vi "SerialUntra.vi"(8 "Cluster":T1, 10 "cluster":T2) -> (1 "OUTPUT":T1)   [LabVIEW 2017, in "libVariable.lvlib" / "LibFunction.lvlib"]
uses:
  LibFunction.lvlib
  controls/QueueControl.ctl
  controls/CommandQueue.ctl
  <vilib>/Platform/TimedLoop/XDataNode/timing_clust.ctl
  <vilib>/Platform/TimedLoop/XDataNode/nitl_modes.ctl
  <vilib>/Platform/TimedLoop/XDataNode/wakeup.ctl
  mWorkToolkit/libSerial/STATEUART.ctl
  controls/state_board_control.ctl
  mWorkToolkit/libSerial/stateSerialUltra.ctl
  <vilib>/Instr/_visa.llb/VISA Flush IO Buffer Mask.ctl
  global/GLOBAL_STATE.vi
  <vilib>/Platform/TimedLoop/XDataNode/XDataNode.xnode
  <vilib>/Platform/TimedLoop/XDataNode/XDNodeRunTimeDep.lvlib
panel:
  out "Data Write":string
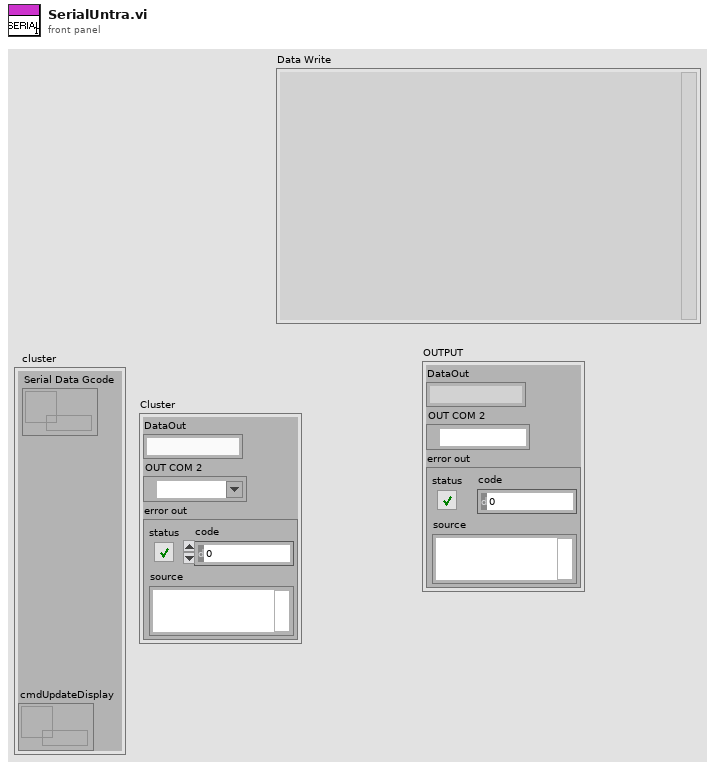
[diagram p1: front panel]
types:
  T1 = cluster{"DataOut":string, "OUT COM 2":refnum<visa-resource-name>, "error out":errorcluster}
  T2 = typedef "QueueControl.ctl" = cluster{"Serial Data Gcode":refnum<queue>, "cmdUpdateDisplay":refnum<queue>}
  T3 = typedef "STATEUART.ctl" = enum16{"INIT", "WRITE", "READ", "CHECKDATA", "IDLE", "STOP"}
  T4 = typedef "XDNodeRunTimeDep.lvlib/timing_clust.ctl" = cluster{"Expected End [f-1]":u64, "Actual End [f-1]":u64, "Finished Late? [f-1]":bool, "Expected End [i-1]":u64, "Actual End [i-1]":u64, "Finished Late? [i-1]":bool, "Expected Start [i]":u64, "Actual Start [i]":u64, "Expected Start [f]":u64, "Actual Start [f]":u64, "Source Name":string, "Structure Name":string, "Period":i64, "Deadline":i64, "Offset":i64, "Start":i64, "Priority":i32, "Timeout":i32, "Mode":T5, "Wakeup Reason":T6, "Error":errorcluster, "Source Type":string, "Secondary Source Type":string, "Global End Time":u64, "Global Start Time":u64, "Frame Duration":u64, "Iteration Duration":u64, "Assigned CPU":i32, "I/O Scan Engine Mode":u32}
  T5 = typedef "XDNodeRunTimeDep.lvlib/nitl_modes.ctl" = enum32{"No Change", "Process missed periods, maintain original phase", "Discard missed periods, maintain original phase", "Process missed periods, ignore original phase", "Discard missed periods, ignore original phase"}
  T6 = typedef "XDNodeRunTimeDep.lvlib/wakeup.ctl" = enum32{"Normal", "Aborted", "Asynchronous wakeup", "Timing source error", "Timed loop error", "Timeout"}
  T7 = typedef "state_board_control.ctl" = enum16{"Running", "Waiting", "Pos", "IDLE"}
  T8 = typedef "stateSerialUltra.ctl" = enum16{"findCOM", "Init", "CheckConnect", "Read", "Write", "exit"}
  T9 = cluster{"DataOut":string, "OUT COM 3":refnum<visa-resource-name>, "error out":errorcluster}
  T10 = cluster{string, "OUT COM 2":refnum<visa-resource-name>, "error IO":errorcluster}
  T11 = cluster{"DataOut":string, "OUT COM 2":refnum<visa-resource-name>, "error out\n":errorcluster}
  T12 = typedef "STATE_MK4DUERETURNSTATE.ctl" = enum16{"Pos", "Config", "Echo", "OK", "Step", "Error"}
  T13 = cluster{"OUTCONFIG":cluster{"StateMcodeConfig":enum16{"M203", "M201", "M92", "M3001"}, "X":dbl, "Y":dbl, "Z":dbl}, "outPOS":cluster{"StatePos":enum16{"Running", "Waiting", "Pos", "IDLE"}, "X":dbl, "Z":dbl, "Y":dbl, "A":dbl, "B":dbl}}
  T14 = cluster{"StateMcodeConfig":enum16{"M203", "M201", "M92", "M3001"}, "X":dbl, "Y":dbl, "Z":dbl}
  T15 = cluster{"StatePos":enum16{"Running", "Waiting", "Pos", "IDLE"}, "X":dbl, "Z":dbl, "Y":dbl, "A":dbl, "B":dbl}
  T16 = cluster{"StatePos":enum16{"Running", "Waiting", "Pos", "IDLE"}, "X":dbl, "Z":dbl, "Y":dbl}
  T17 = typedef "VISA Flush IO Buffer Mask.ctl" = u16
  T18 = cluster{"TIMEOUT_CONNECT":u32, "TIMEOUT_SENDCHECK":u32}
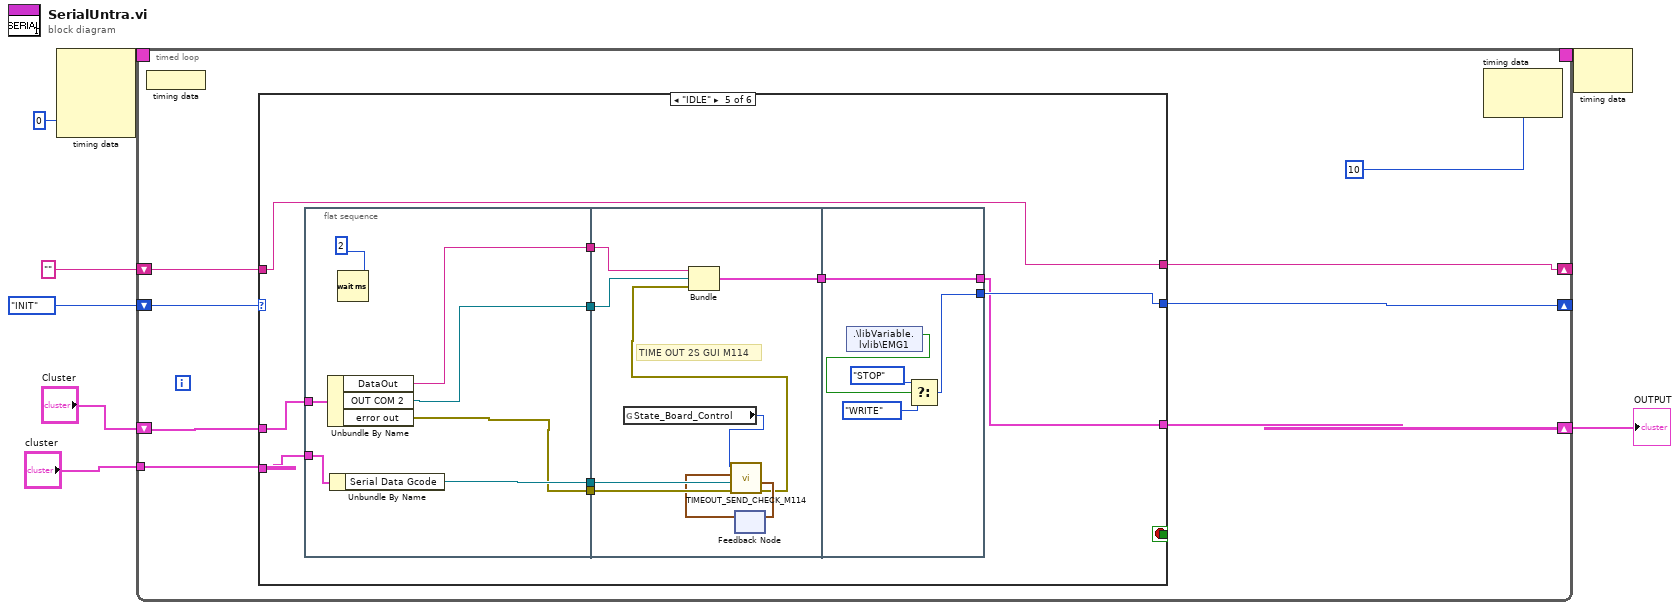
[diagram p0: block diagram]
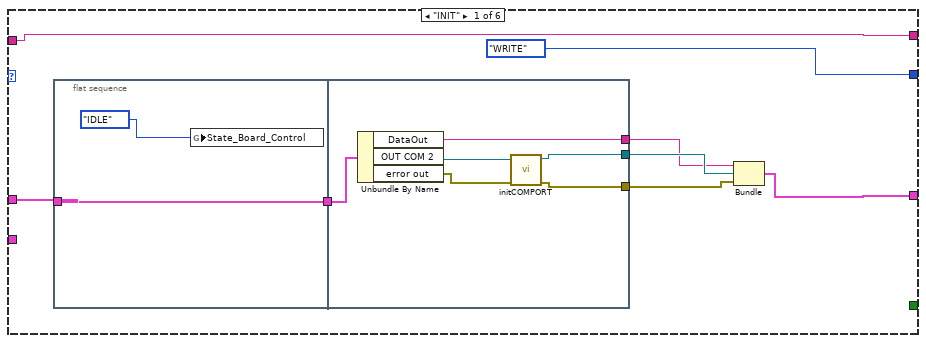
[diagram p2: hidden frame]
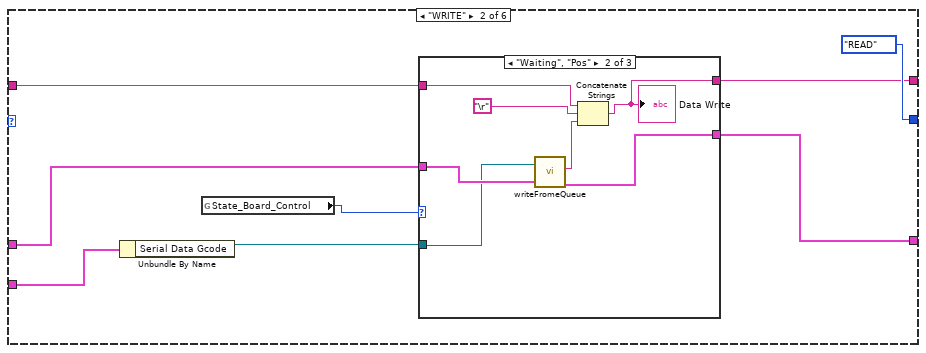
[diagram p3: hidden frame]
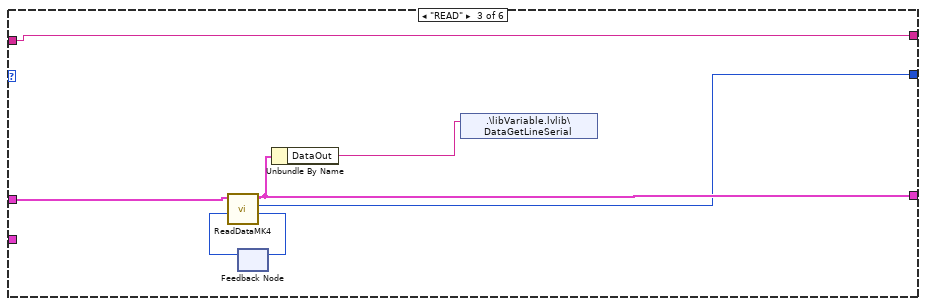
[diagram p6: hidden frame]
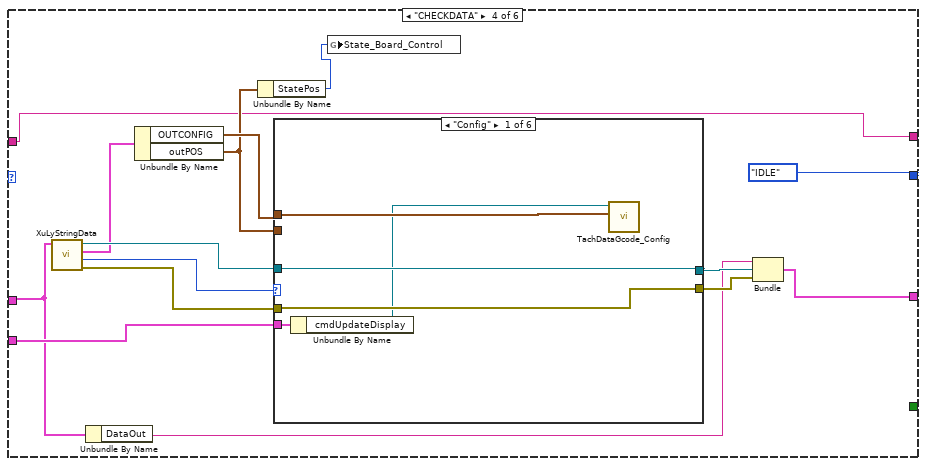
[diagram p7: hidden frame]
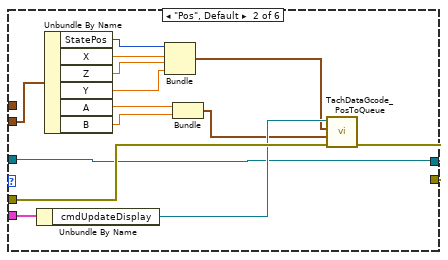
[diagram p8: hidden frame]
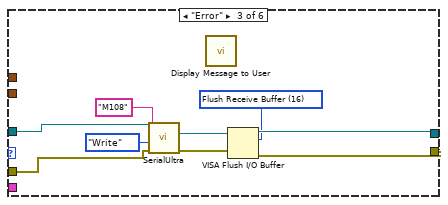
[diagram p9: hidden frame]
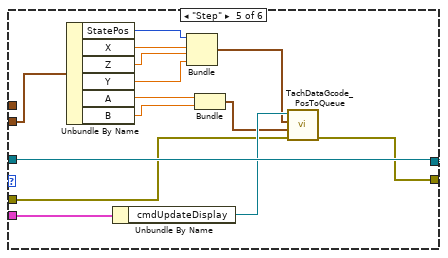
[diagram p11: hidden frame]
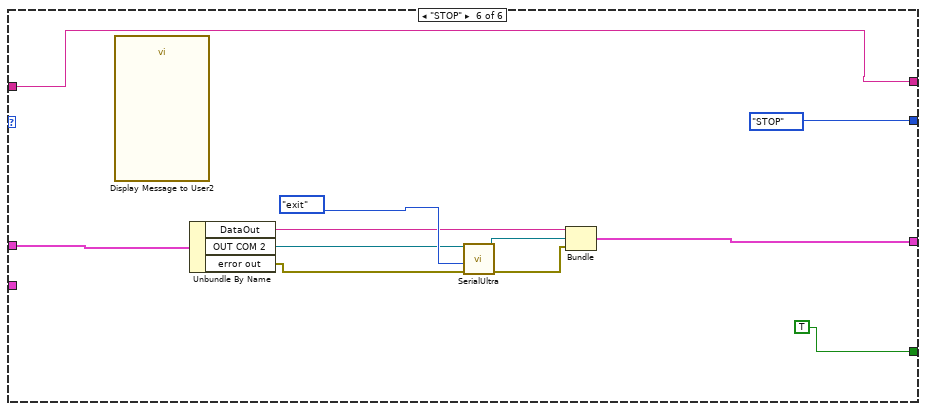
[diagram p13: hidden frame]
diagram:
  n1 = node-c288(0 ("Processor")) -> (w8:T4)  [unwired: 3 in]
  n2 = timed-loop {
    shift-right: [w14] -> _
    shift-left: STATEUART."INIT" -> [w17]
    shift-right: [w13] -> w2
    shift-left: "Cluster" -> [w15]
    timing: w8 -> [_]
    timing-out: [_] -> w7
    tunnel: "cluster" -> [w16]
    shift-right: [w9] -> _
    shift-left: "" -> [w10]
    stop <- w11 stop-if-true
    n3 = node-c288() -> ()  [unwired: 1 in]
    n4 = case shown="\"IDLE\"" w17 {
      tunnel: [STATEUART."WRITE" STATEUART."READ" w54 STATEUART."IDLE" w125 STATEUART."STOP"] -> w14
      tunnel: w15 -> [w22 w40 w59 w63 w130 w155]
      tunnel: [w20 w38 w56 w64 w123 w154] -> w13
      tunnel: w16 -> [_ w41 _ w68 w122 _]
      tunnel: [_ _ _ _ _ TRUE] -> w11
      tunnel: w10 -> [w18 w36 w53 w61 w121 w152]
      tunnel: [w18 w35 w53 w61 w121 w152] -> w9
      frame "INIT" {
        n5 = flat-sequence {
          tunnel: [w27] -> w25
          tunnel: w22 -> [w27]
          tunnel: w25 -> [w30]
          tunnel: [w31] -> w19
          tunnel: [w29] -> w23
          tunnel: [w28] -> w24
          frame #0 {
            n6 = global write "GLOBAL_STATE.vi" "State_Board_Control"(state_board_control."IDLE" ("state_board_STM1")) -> ()
          }
          frame #1 {
            n7 = Unbundle By Name(w30) -> ("DataOut"=w31:string, "OUT COM 2"=w33:refnum<visa-resource-name>, "error out"=w32:errorcluster)
            n8 = call "initCOMPORT.vi"("error IO"=w32, "OUT COM 2"=w33) -> ("error out"=w29:errorcluster, "OUT COM 3"=w28:refnum<visa-resource-name>)  [unwired: 8 in]
          }
        }
        n9 = Bundle("DataOut"=w19, "OUT COM 3"=w24, "error out"=w23) -> (w20:T9)  [unwired: 1 in]
      }
      frame "WRITE" {
        n10 = Unbundle By Name(w41) -> ("Serial Data Gcode"=w39:refnum<queue>)
        n11 = global read "GLOBAL_STATE.vi" "State_Board_Control"() -> (w34:T7)
        n12 = case shown="\"Waiting\", \"Pos\"" w34 {
          tunnel: w40 -> [w43 w50 w52]
          tunnel: w39 -> [_ w49 _]
          tunnel: [w43 w48 w52] -> w38
          tunnel: w36 -> [w42 w47 w51]
          tunnel: [w42 w46 w51] -> w35
          frame "Running", Default {
          }
          frame "Waiting", "Pos" {
            n13 = call "writeFromeQueue.vi"("queue"=w49, "Cluster"=w50) -> ("output cluster"=w48:T10, "Data Write"=w45:string)  [unwired: 7 in, 1 out]
            n14 = Concatenate Strings(w47, "\r", w45) -> (w46:string)
            "Data Write" <- w46
          }
          frame "IDLE" {
          }
        }
      }
      frame "READ" {
        n15 = feedback #1() -> (w57:u32)  [unwired: 1 in]
        n16 = call "ReadDataMK4.vi"("millisecondIN"=w57, "input cluster"=w59) -> ("millisecondOUT"=w58:u32, "STATEUART"=w54:T3, "Cluster"=w56:T11)  [unwired: 7 in]
        n17 = feedback-in #1(w58) -> ()
        n18 = Unbundle By Name(w56) -> ("DataOut"=w55:string)
        n19 = shared-variable ".\\libVariable.lvlib\\DataGetLineSerial"(w55) -> ()  [unwired: 1 in, 1 out]
      }
      frame "CHECKDATA" {
        n20 = call "XuLyStringData.vi"("input cluster"=w63) -> ("error out"=w69:errorcluster, "Return State"=w70:T12, "output cluster 2"=w65:T13, "OUT COM 2"=w71:refnum<visa-resource-name>)  [unwired: 3 in]
        n21 = Unbundle By Name(w63) -> ("DataOut"=w62:string)
        n22 = Unbundle By Name(w65) -> ("OUTCONFIG"=w67:T14, "outPOS"=w66:T15)
        n23 = Unbundle By Name(w66) -> ("StatePos"=w60:enum16{"Running", "Waiting", "Pos", "IDLE"})
        n24 = case shown="\"Config\"" w70 {
          tunnel: [w76 w91 w96 w103 w114 w119] -> w73
          tunnel: w69 -> [w76 w92 w94 w103 w115 w119]
          tunnel: w71 -> [w78 w89 w102 w104 w118 w120]
          tunnel: [w78 w89 w97 w104 w118 w120] -> w72
          tunnel: w68 -> [w77 w93 _ _ w117 _]
          tunnel: w67 -> [w79 _ _ _ _ _]
          tunnel: w66 -> [_ w88 _ _ w108 _]
          frame "Config" {
            n25 = Unbundle By Name(w77) -> ("cmdUpdateDisplay"=w75:refnum<queue>)
            n26 = call "TachDataGcode_Config.vi"("OUTCONFIG"=w79, "queue out"=w75) -> ()  [unwired: 10 in]
          }
          frame "Pos", Default {
            n27 = Unbundle By Name(w93) -> ("cmdUpdateDisplay"=w90:refnum<queue>)
            n28 = Unbundle By Name(w88) -> ("StatePos"=w87:enum16{"Running", "Waiting", "Pos", "IDLE"}, "X"=w86:dbl, "Z"=w85:dbl, "Y"=w84:dbl, "A"=w82:dbl, "B"=w81:dbl)
            n29 = Bundle("StatePos"=w87, "X"=w86, "Z"=w85, "Y"=w84) -> (w83:T16)  [unwired: 1 in]
            n30 = Bundle("A"=w82, "B"=w81) -> (w80:cluster{"A":dbl, "B":dbl})  [unwired: 1 in]
            n31 = call "TachDataGcode_PosToQueue.vi"("error in (no error)"=w92, "OUTDGREES"=w80, "outPOS"=w83, "queue out"=w90) -> ("error out"=w91:errorcluster)  [unwired: 7 in]
          }
          frame "Error" {
            w95 = T17 16 items=["Flush Receive Buffer"=16, "Write Transmit Buffer to Device"=32, "Flush Receive Buffer (No I/O)"=64, "Flush Transmit Buffer"=128] ("Mask")
            n32 = call "SerialUltra.vi"("error in"=w94, "State"=stateSerialUltra."Write", "Data Write"="M108", "IN COM"=w102) -> ("error out"=w98:errorcluster, "OUT COM 2"=w99:refnum<visa-resource-name>)  [unwired: 3 in, 3 out]
            n33 = call "Display Message to User"() -> ()  [unwired: 10 in, 2 out]
            n34 = VISA Flush I/O Buffer(VISA resource name=w99, mask (16)=w95, error in (no error)=w98) -> (VISA resource name out=w97:refnum<visa-resource-name>, error out=w96:errorcluster)
          }
          frame "OK" {
          }
          frame "Step" {
            (unwired) ""
            n35 = Unbundle By Name(w108) -> ("StatePos"=w106:enum16{"Running", "Waiting", "Pos", "IDLE"}, "X"=w113:dbl, "Z"=w112:dbl, "Y"=w111:dbl, "A"=w110:dbl, "B"=w109:dbl)
            n36 = Unbundle By Name(w117) -> ("cmdUpdateDisplay"=w116:refnum<queue>)
            n37 = Bundle("StatePos"=w106, "X"=w113, "Z"=w112, "Y"=w111) -> (w107:T16)  [unwired: 1 in]
            n38 = Bundle("A"=w110, "B"=w109) -> (w105:cluster{"A":dbl, "B":dbl})  [unwired: 1 in]
            n39 = call "TachDataGcode_PosToQueue.vi"("error in (no error)"=w115, "OUTDGREES"=w105, "outPOS"=w107, "queue out"=w116) -> ("error out"=w114:errorcluster)  [unwired: 7 in]
          }
          frame "Echo" {
          }
        }
        n40 = global write "GLOBAL_STATE.vi" "State_Board_Control"(w60) -> ()
        n41 = Bundle("DataOut"=w62, "OUT COM 2"=w72, "error out"=w73) -> (w64:T1)  [unwired: 1 in]
      }
      frame "IDLE" {
        n42 = flat-sequence {
          tunnel: w122 -> [w137]
          tunnel: w130 -> [w136]
          tunnel: [w135] -> w129
          tunnel: [w134] -> w128
          tunnel: [w131] -> w127
          tunnel: [w132] -> w126
          tunnel: w129 -> [w142]
          tunnel: w128 -> [w141]
          tunnel: w127 -> [w146]
          tunnel: w126 -> [w145]
          tunnel: [w139] -> w124
          tunnel: [w149] -> w125
          tunnel: [w147] -> w123
          tunnel: w124 -> [w147]
          frame #0 {
            n43 = Unbundle By Name(w136) -> ("DataOut"=w135:string, "OUT COM 2"=w134:refnum<visa-resource-name>, "error out"=w131:errorcluster)
            n44 = Unbundle By Name(w137) -> ("Serial Data Gcode"=w132:refnum<queue>)
            n45 = Wait (ms)(milliseconds to wait=u32 2) -> ()  [unwired: 1 out]
          }
          frame #1 {
            # "TIME OUT 2S GUI M114"
            n46 = global read "GLOBAL_STATE.vi" "State_Board_Control"() -> (w138:T7)
            n47 = feedback #2() -> (w143:T18)  [unwired: 1 in]
            n48 = call "TIMEOUT_SEND_CHECK_M114.vi"("error IN"=w146, "Serial Data Gcode"=w145, "IN TIME"=w143, "STATE BOARD"=w138) -> ("error out"=w140:errorcluster, "OUT TIME"=w144:T18)  [unwired: 6 in]
            n49 = Bundle("DataOut"=w142, "OUT COM 2"=w141, "error out"=w140) -> (w139:T1)  [unwired: 1 in]
            n50 = feedback-in #2(w144) -> ()
          }
          frame #2 {
            n51 = shared-variable ".\\libVariable.lvlib\\EMG1"() -> (w148:bool)  [unwired: 1 in, 1 out]
            n52 = Select(t=STATEUART."STOP", s=w148, f=STATEUART."WRITE") -> (s? t:f=w149:T3)
          }
        }
      }
      frame "STOP" {
        (unwired) TRUE
        n53 = call "Display Message to User2"() -> ()  [unwired: 10 in, 2 out]
        n54 = Unbundle By Name(w155) -> ("DataOut"=w157:string, "OUT COM 2"=w160:refnum<visa-resource-name>, "error out"=w159:errorcluster)
        n55 = call "SerialUltra.vi"("error in"=w159, "State"=stateSerialUltra."exit", "IN COM"=w160) -> ("error out"=w156:errorcluster, "OUT COM 2"=w158:refnum<visa-resource-name>)  [unwired: 4 in, 3 out]
        n56 = Bundle("DataOut"=w157, "OUT COM 2"=w158, "error out"=w156) -> (w154:T11)  [unwired: 1 in]
      }
    }
    n57 = node-c288(i64 10 ("Period")) -> ()  [unwired: 1 in, 1 out]
  }
  "OUTPUT" <- w2
  n58 = node-c288(w7) -> ()  [unwired: 1 out]
